vi "_067.vi"() -> ()   [LabVIEW 2024]
panel:
  out "Iteration":i32
  in  "OK Button":bool
  # "Avoiding front panel polling :"
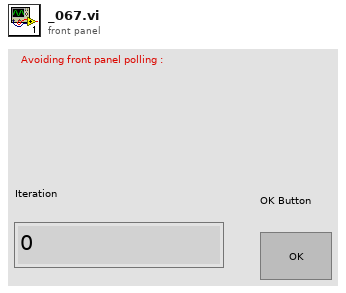
[diagram p1: front panel]
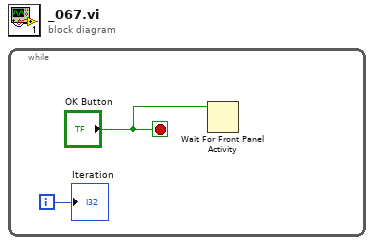
[diagram p0: block diagram]
diagram:
  n1 = while {
    i -> [w2]
    stop <- "OK Button" stop-if-true
    n2 = Wait For Front Panel Activity(3:"OK Button") -> ()  [unwired: 2 in, 1 out]
    "Iteration" <- w2
  }
